vi "filter.test.AddOrder.and.OrderExecuted.Pass.Through.vi"() -> ()   [LabVIEW 2022 SP3]
uses:
  fpga/common/orderbook.command.ctl
  fpga/common/orderbook.command.type.ctl
panel:
  out "GetState":u64[](array[numeric]) format="%.0x"
  in  "Expected.GetState":u64[](array[numeric])=[4702127773838221344, 176, 6076284164848492576, 177, 32, 20000, 48, 20000] format="%.0x"
  out "error out":errorcluster
  out "Debug":u64[](array[numeric]) format="%.0x"
  out "Passed":bool
  out "OrderBook.Commands.out":T1[](array[typedef]) {"Side (U8)" format="%.0x"; "Order Id (U64)" format="%.0x"; "Symbol (U64)" format="%.0x"}
  in  "OrderBook.Commands.in":T1[](array[typedef])=[{"OrderBook Command.Type"=enum."AddOrder", "Side (U8)"=66, "Order Id (U64)"=48, "Quantity (U32)"=20000, "Symbol (U64)"=4702127773838221344, "Price (U64)"=9050, "Executed Quantity (U32)"=0, "Canceled Quantity (U32)"=0, "Remaining Quantity (U32)"=0, "Seconds (U64)"=0, "Nanoseconds (U64)"=0}, {"OrderBook Command.Type"=enum."OrderExecuted", "Side (U8)"=66, "Order Id (U64)"=48, "Quantity (U32)"=20000, "Symbol (U64)"=0, "Price (U64)"=9050, "Executed Quantity (U32)"=0, "Canceled Quantity (U32)"=0, "Remaining Quantity (U32)"=0, "Seconds (U64)"=0, "Nanoseconds (U64)"=0}, {"OrderBook Command.Type"=enum."AddOrder", "Side (U8)"=66, "Order Id (U64)"=32, "Quantity (U32)"=20000, "Symbol (U64)"=6076284164848492576, "Price (U64)"=9050, "Executed Quantity (U32)"=0, "Canceled Quantity (U32)"=0, "Remaining Quantity (U32)"=0, "Seconds (U64)"=0, "Nanoseconds (U64)"=0}] {"Side (U8)" format="%.0x"; "Order Id (U64)" format="%.0x"; "Symbol (U64)" format="%.0x"}
  in  "Watch.List":string[](array[string])=["AAPL", "TSLA"]
  in  "Expected OrderBook.Commands":T1[](array[typedef])=[{"OrderBook Command.Type"=enum."AddOrder", "Side (U8)"=66, "Order Id (U64)"=48, "Quantity (U32)"=20000, "Symbol (U64)"=4702127773838221344, "Price (U64)"=9050, "Executed Quantity (U32)"=0, "Canceled Quantity (U32)"=0, "Remaining Quantity (U32)"=0, "Seconds (U64)"=0, "Nanoseconds (U64)"=0}, {"OrderBook Command.Type"=enum."OrderExecuted", "Side (U8)"=66, "Order Id (U64)"=48, "Quantity (U32)"=20000, "Symbol (U64)"=0, "Price (U64)"=9050, "Executed Quantity (U32)"=0, "Canceled Quantity (U32)"=0, "Remaining Quantity (U32)"=0, "Seconds (U64)"=0, "Nanoseconds (U64)"=0}, {"OrderBook Command.Type"=enum."AddOrder", "Side (U8)"=66, "Order Id (U64)"=32, "Quantity (U32)"=20000, "Symbol (U64)"=6076284164848492576, "Price (U64)"=9050, "Executed Quantity (U32)"=0, "Canceled Quantity (U32)"=0, "Remaining Quantity (U32)"=0, "Seconds (U64)"=0, "Nanoseconds (U64)"=0}] {"Side (U8)" format="%.0x"; "Order Id (U64)" format="%.0x"; "Symbol (U64)" format="%.0x"}
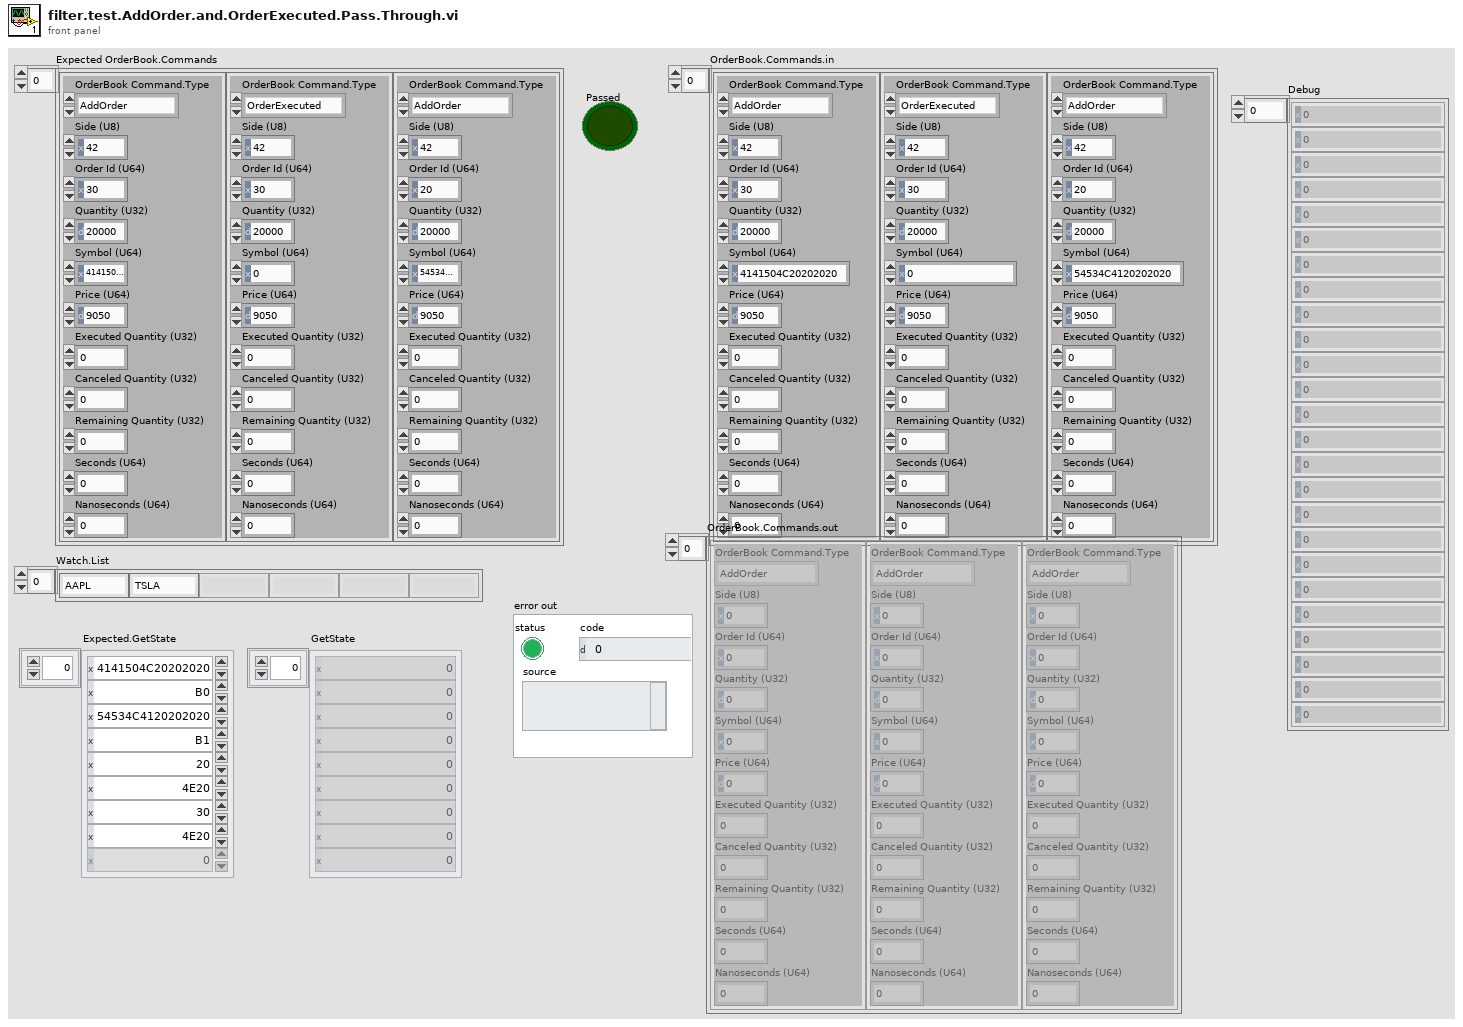
[diagram p1: front panel]
types:
  T1 = typedef "orderbook.command.ctl" = cluster{"OrderBook Command.Type":T2, "Side (U8)":u8, "Order Id (U64)":u64, "Quantity (U32)":u32, "Symbol (U64)":u64, "Price (U64)":u64, "Executed Quantity (U32)":u32, "Canceled Quantity (U32)":u32, "Remaining Quantity (U32)":u32, "Seconds (U64)":u64, "Nanoseconds (U64)":u64}
  T2 = typedef "orderbook.command.type.ctl" = enum16{"Time", "AddOrder", "OrderExecuted", "OrderExecutedAtPrice", "ReduceSize", "ModifyOrder", "DeleteOrder", "Get.State", "Get.All.Orders", "Get.Top"}
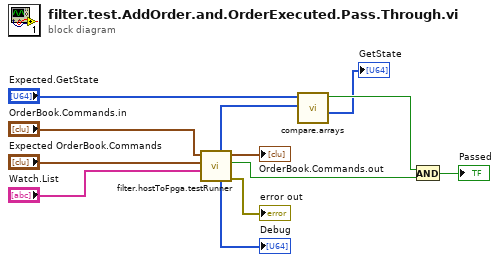
[diagram p0: block diagram]
diagram:
  n1 = call "filter.hostToFpga.testRunner.vi"("Watch.List"="Watch.List", "Expected OrderBook.Command[]"="Expected OrderBook.Commands", "OrderBook.Commands.in"="OrderBook.Commands.in") -> ("error out"=→"error out":errorcluster, "Passed"=w4:bool, "OrderBook.Commands.out"=→"OrderBook.Commands.out":T1[], "Debug"=→"Debug":u64[], "GetState"=w5:u64[])  [unwired: 3 in, 1 out]
  n2 = call "compare.arrays.vi"("Actual"=w5, "Expected"="Expected.GetState") -> ("Actual.Out"=→"GetState":u64[], "Full.Match"=w3:bool)  [unwired: 7 in, 1 out]
  n3 = And(x=w3, y=w4) -> (x .and. y?=→"Passed":bool)
